vi "Plot and Render 3D with rotation.vi"() -> ()   [LabVIEW 2010]
uses:
  <vilib>/Math Plots/3D Math Plots/3D Scatter/3D Scatter XCtrl/3D Scatter.xctl
  <vilib>/Math Plots/3D Math Plots/3D Scatter/3D Scatter Datatype/3D Scatter Datatype.lvclass
  <vilib>/Analysis/Matrix/Datatypes/RealMatrix.ctl
  <vilib>/Utility/miscctls.llb/LVRGBAColorTypeDef.ctl
  <vilib>/Math Plots/3D Math Plots/3D Scatter/3D Scatter Datatype/Public/Plot Helper (Vector).vi
  <vilib>/Analysis/baseanly.llb/A x Vector.vi
  <vilib>/Analysis/NI_AALBase.lvlib
  <vilib>/Analysis/Matrix/NI_Matrix.lvlib
panel:
  out "Rotated Cell":dbl[][](array[numeric])=[[1.0, 0.0, 0.0], [0.0, -0.9814838910603481, 0.1915446986711951], [0.0, -0.1915446986711951, -0.9814838910603481], [-1.0, 0.0, 0.0], [0.0, 0.9814838910603481, -0.1915446986711951], [0.0, 0.1915446986711951, 0.9814838910603481]]
  in  "Rotation Angle":dbl(slide)=168.95705521472394 scale=0.0..360.0
  out "X Rotation Matrix":T1=[[1.0, 0.0, 0.0], [0.0, -0.9814838910603481, -0.1915446986711951], [0.0, 0.1915446986711951, -0.9814838910603481]]
  out "Scene Display":refnum<vi>(3d-picture)
  out "3D Scatter":refnum<class "3D Plot Datatype.lvclass">[](xcontrol)
  in  "Bravais Lattice C":dbl[](array[numeric])
  in  "Bravais Lattice B":dbl[](array[numeric])
  in  "Bravais Lattice A":dbl[](array[numeric])
  in  "Original Unit Cell":dbl[][](array[numeric])=[[1.0, 0.0, 0.0], [0.0, 1.0, 0.0], [0.0, 0.0, 1.0], [-1.0, 0.0, 0.0], [0.0, -1.0, 0.0], [0.0, 0.0, -1.0]]
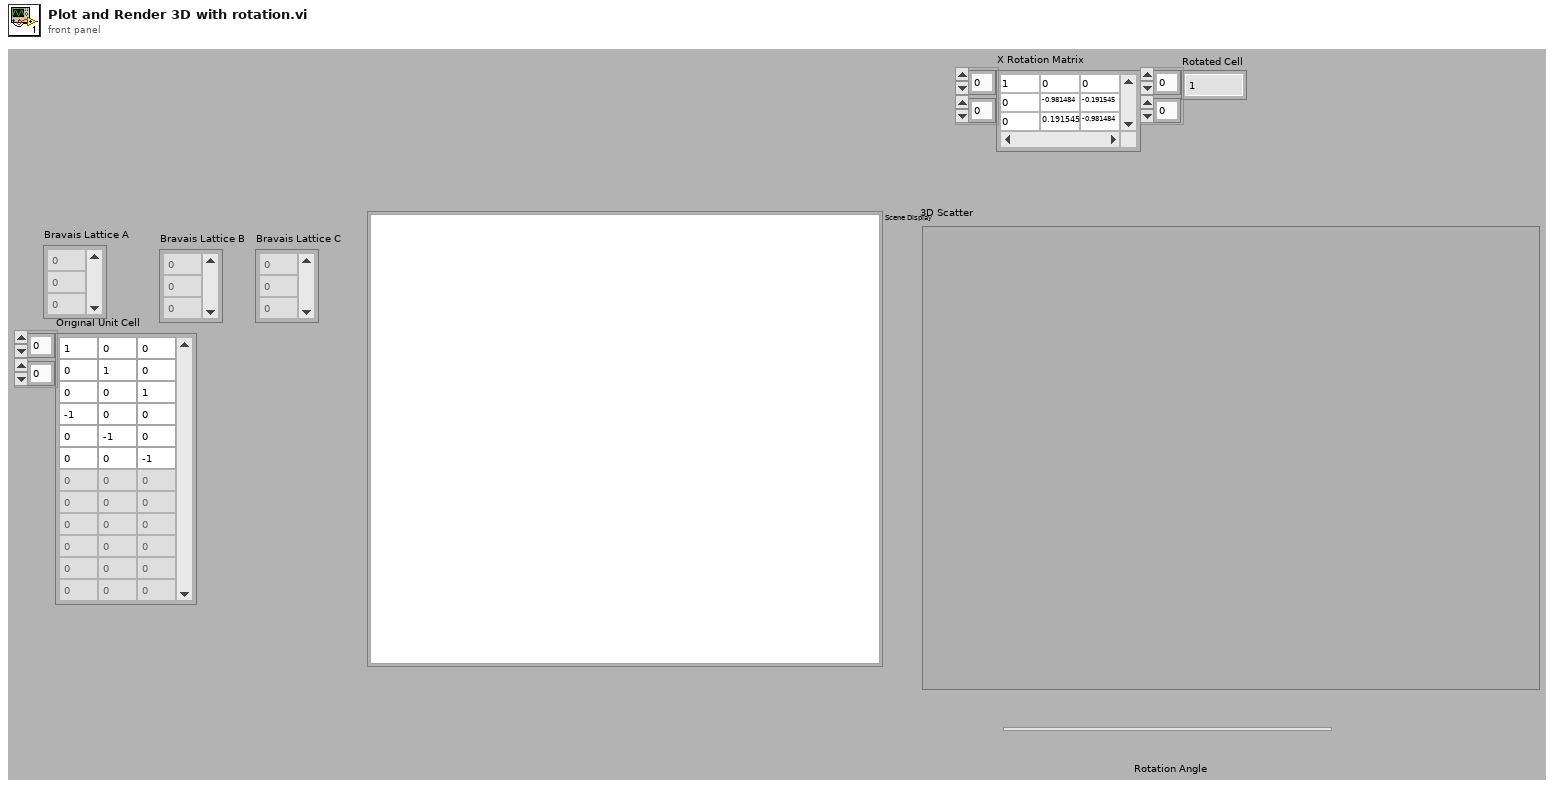
[diagram p1: front panel]
types:
  T1 = typedef "NI_Matrix.lvlib/RealMatrix.ctl" = dbl[][]
  T2 = typedef "LVRGBAColorTypeDef.ctl" = cluster{"Red":sgl, "Green":sgl, "Blue":sgl, "Alpha":sgl}
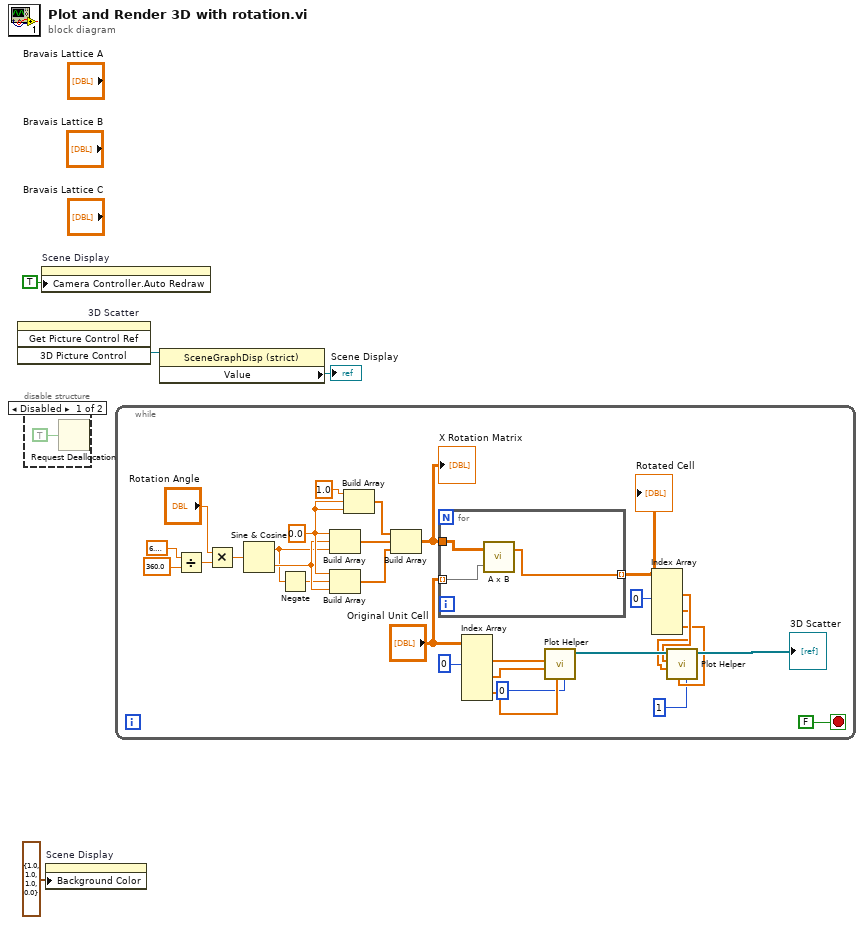
[diagram p0: block diagram]
diagram:
  n1 = invoke on="3D Scatter" class="3D Scatter (strict)" method="Get Picture Control Ref"() -> ("3D Picture Control"=w4:refnum<vi>)  [unwired: 4 in, 3 out]
  n2 = disable-structure shown="Disabled" {
    frame Disabled {
      n3 = Request Deallocation(TRUE ("flag")) -> ()
    }
    frame Enabled {
    }
  }
  n4 = property on="Scene Display" class="SceneGraphDisp (strict)"("Camera Controller.Auto Redraw"=TRUE ("Camera Controller:Auto Redraw")) -> ()  [unwired: 2 in, 2 out]
  n5 = property on="Scene Display" class="SceneGraphDisp (strict)"("Background Color"=T2 {"Red"=1.0, "Green"=1.0, "Blue"=1.0, "Alpha"=0.0}) -> ()  [unwired: 2 in, 2 out]
  n6 = while {
    stop <- FALSE stop-if-true
    w25 = 0.0 ("element")
    n7 = Divide(x=6.283185307179586, y=360.0) -> (x/y=w20:dbl)
    n8 = Multiply(x="Rotation Angle", y=w20) -> (x*y=w19:dbl)
    n9 = Sine & Cosine(0:w19) -> (1:w15:dbl, 2:w24:dbl)
    n10 = Negate(x=w15) -> (-x=w23:dbl)
    n11 = Build Array(w25, w24, w15) -> (w16:dbl[])
    n12 = Build Array(w25, w23, w24) -> (w14:dbl[])
    n13 = Build Array(1.0 ("element"), w25, w25) -> (w26:dbl[])
    n14 = Build Array(w26, w16, w14) -> (w17:T1)
    "X Rotation Matrix" <- w17
    n15 = for {
      tunnel: "Original Unit Cell" -> [w36] mode=indexing
      tunnel: w17 -> [w37]
      tunnel: [w35] -> w13 mode=indexing
      n16 = call-poly <vilib>:"A x B.vi"("Vector"=w36, "A"=w37) -> ("A x Vector"=w35:dbl[])  [unwired: 1 out]
    }
    "Rotated Cell" <- w13
    n17 = Index Array(array="Original Unit Cell", index (col) #1=0 ("disabled index (col)")) -> (element #1=w33:dbl[], element #2=w32:dbl[], element #3=w31:dbl[])  [unwired: 5 in]
    n18 = call-poly <vilib>:"Plot Helper.vi"("Plot ID"=0, "z vector"=w31, "y vector"=w32, "x vector"=w33) -> ("3D Plot lvclass Array out"=w30:refnum<class "3D Plot Datatype.lvclass">[])  [unwired: 2 in, 5 out]
    n19 = Index Array(array=w13, index (col) #1=0 ("disabled index (col)")) -> (element #1=w11:dbl[], element #2=w10:dbl[], element #3=w9:dbl[])  [unwired: 5 in]
    n20 = call-poly <vilib>:"Plot Helper.vi"("Plot ID"=1, "z vector"=w9, "y vector"=w10, "x vector"=w11, "3D Plot lvclass Array in"=w30) -> ("3D Plot lvclass Array out"=→"3D Scatter":refnum<class "3D Plot Datatype.lvclass">[])  [unwired: 1 in, 5 out]
  }
  n21 = property class="SceneGraphDisp (strict)"(reference=w4) -> ("Value"=→"Scene Display":refnum<vi>)  [unwired: 1 in, 2 out]
